vi "GenerateUniqueFilename -- V2.vi"(5 "Index digits":i32=3, 6 "new suffix":string="_tdo_", 7 "format string":string="%d", 8 "Error In":errorcluster, 9 "ovewrite file?":bool=TRUE, 10 "dot name suffix":string=".dat", 11 "file Path IN":path=path "/Users/arkadyshekhter/Desktop/gdrive/data/Vikram&Shiva&Zoltan--Aug2025/August_2025/082225/p_c4_012_082225.tdms") -> (0 "Error Out":errorcluster, 3 "file Path OUT":path=path "/Users/arkadyshekhter/Desktop/gdrive/data/Vikram&Shiva&Zoltan--Aug2025/August_2025/082225/p_c4_012_082225_tdo_0.dat/p_c4_012_082225_tdo_1.dat")   [LabVIEW 2021]
uses:
  filename-action.ctl
panel:
  out "Any file exists?":bool
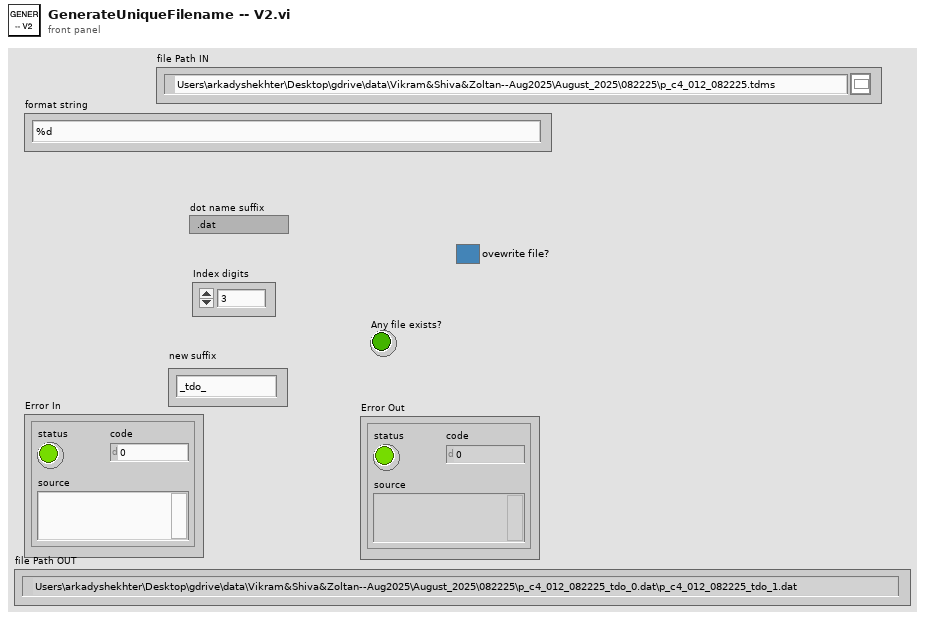
[diagram p1: front panel]
types:
  T1 = typedef "filename-action.ctl" = enum16{"rewrite", "parse", "force pattern", "uniquenum", "get T", "get B", "get ind", "get deg", "get name", "get folder", "get extension", "get basename", "get side", "get setof", "getID", "getIDStock", "remove prefix", "get36thing", "getplain", "getvproj", "getIDStanf"}
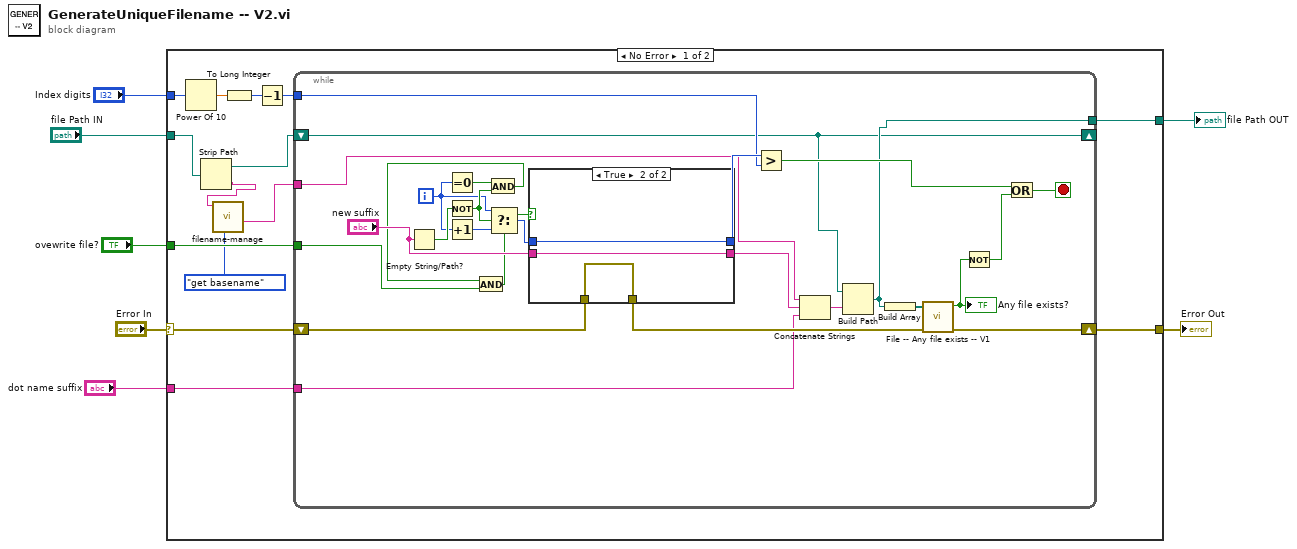
[diagram p0: block diagram]
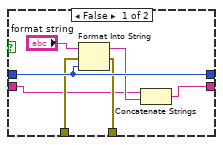
[diagram p2: hidden frame]
diagram:
  n1 = case shown="No Error" "Error In" {
    selector: "Error In" -> [w20 w58]
    tunnel: [w21 w58] -> w6
    tunnel: "Index digits" -> [w19 _]
    tunnel: "file Path IN" -> [w15 _]
    tunnel: [w8 _] -> w3
    tunnel: "ovewrite file?" -> [w13 _]
    tunnel: "dot name suffix" -> [w10 _]
    frame No Error {
      n2 = Power Of 10(x=w19) -> (10^x=w18:dbl)
      n3 = Strip Path(path=w15) -> (stripped path=w14:path, name=w12:string)
      n4 = call "filename-manage.vi"("filename-action"=filename-action."get basename", "file name IN"=w12) -> ("string OUT"=w9:string)  [unwired: 7 in, 2 out]
      n5 = To Long Integer(number=w18) -> (32bit integer=w17:i32)
      n6 = Decrement(x=w17) -> (x-1=w16:i32)
      n7 = while {
        shift-right: [w43] -> w21
        shift-left: w20 -> [w32]
        tunnel: w16 -> [w35]
        tunnel: w9 -> [w28]
        shift-right: [w22] -> _
        shift-left: w14 -> [w22]
        tunnel: w13 -> [w26]
        tunnel: w10 -> [w24]
        tunnel: [w23] -> w8
        i -> [w37]
        stop <- w45 stop-if-true
        n8 = Empty String/Path?(string/path="new suffix") -> (empty?=w41:bool)
        n9 = Equal To 0?(x=w37) -> (x = 0?=w39:bool)
        n10 = Not(x=w41) -> (.not. x?=w38:bool)
        n11 = Increment(x=w37) -> (x+1=w36:i32)
        n12 = And(x=w39, y=w38) -> (x .and. y?=w27:bool)
        n13 = And(x=w27, y=w26) -> (x .and. y?=w25:bool)
        n14 = Select(t=w37, s=w38, f=w36) -> (s? t:f=w42:i32)
        n15 = case shown="True" w25 {
          tunnel: [w48 w56] -> w47
          tunnel: [w53 w57] -> w46
          tunnel: w42 -> [w53 w57]
          tunnel: "new suffix" -> [w49 w56]
          tunnel: w32 -> [w52 w55]
          tunnel: [w51 w55] -> w31
          frame False {
            n16 = Format Into String(format string="format string", error in=w52, w53) -> (resulting string=w50:string, error out=w51:errorcluster)  [unwired: 1 in]
            n17 = Concatenate Strings(w49, w50) -> (w48:string)
          }
          frame True {
          }
        }
        n18 = Greater?(x=w46, y=w35) -> (0:w33:bool)
        n19 = Concatenate Strings(w28, w47, w24) -> (w30:string)
        n20 = Build Path(base path=w22, name or relative path=w30) -> (appended path=w23:path)
        n21 = Build Array(w23) -> (w29:path[])
        n22 = call "File -- Any file exists -- V1.vi"("Error In"=w31, "Files"=w29) -> ("Error Out"=w43:errorcluster, "Any file exists?"=w44:bool)  [unwired: 8 in]
        "Any file exists?" <- w44
        n23 = Not(x=w44) -> (.not. x?=w34:bool)
        n24 = Or(x=w33, y=w34) -> (x .or. y?=w45:bool)
      }
    }
    frame Error {
    }
  }
  "Error Out" <- w6
  "file Path OUT" <- w3
